vi "Fast_spectrum_analyzer_diag.vi"(8 "error in (no error)":errorcluster, 9 "mean":dbl, 10 "Waveform":waveform(dbl), 11 "Frequency":dbl) -> (0 "error out":errorcluster, 1 "MLD SA (mV/V)":dbl, 2 "Spectrum (mV/V)":cluster{"f0":dbl, "df":dbl, "magnitude":dbl[]}(graph), 3 "1f Peak (mv/V)":dbl)   [LabVIEW 2013]
uses:
  <vilib>/express/express analysis/Spectral/Block/exnSpectralBlock spectral measurements RMS poly.vi
  <vilib>/express/express analysis/Spectral/Block/exnSpectralBlock spectral measurements RMS WFM.vi
  <vilib>/express/express analysis/Spectral/XNode/ExpressSpectralMeasurementsBlockNode.xnode
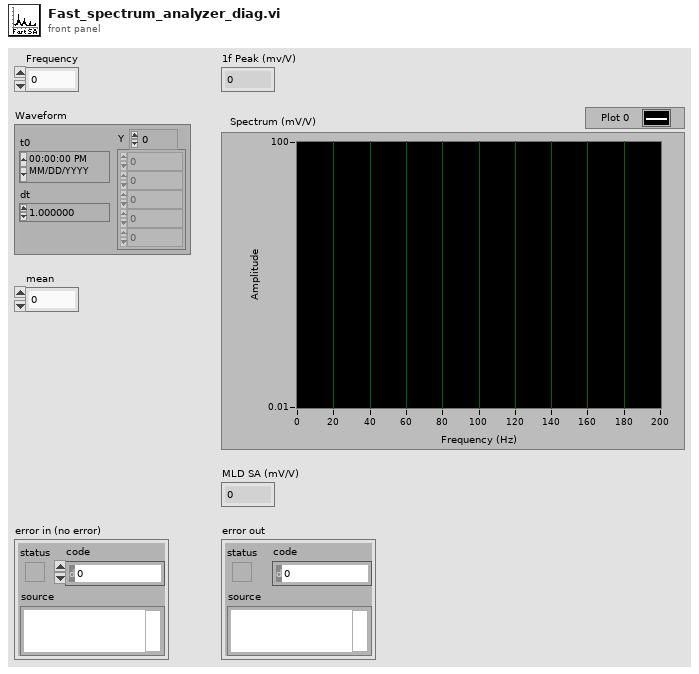
[diagram p1: front panel]
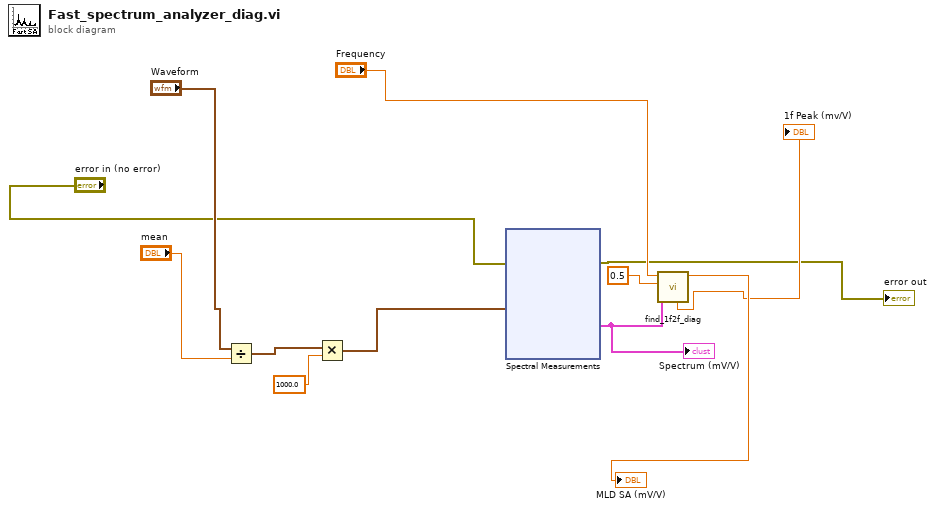
[diagram p0: block diagram]
diagram:
  n1 = Divide(x="Waveform", y="mean") -> (x/y=w6:waveform(dbl))
  n2 = Multiply(x=w6, y=1000.0) -> (x*y=w5:waveform(dbl))
  n3 = xnode "Spectral Measurements"("Signals"=w5, "error in (no error)"="error in (no error)") -> ("FFT - (RMS)"=w11:cluster{"f0":dbl, "df":dbl, "magnitude":dbl[]}, "error out"=→"error out":errorcluster)  [unwired: 1 out]
  "Spectrum (mV/V)" <- w11
  n4 = call "find_1f2f_diag.vi"("FFT - (RMS)"=w11, "Peak FWHM"=0.5, "Central Frequency"="Frequency") -> ("2f Peak Amplitude (mVrms/Vdc)"=→"MLD SA (mV/V)":dbl, "1f Peak Amplitude(mVrms/Vdc)"=→"1f Peak (mv/V)":dbl)  [unwired: 4 in, 3 out]
